vi "10 - colour keying.vi"() -> ()   [LabVIEW 2015]
uses:
  Libraries/LibSDL2 Wrapper/Controls/Init Flags.ctl
  Libraries/LibSDL2 Wrapper/Controls/NULL.ctl
  Libraries/LibSDL2 Wrapper/Controls/Rectangle.ctl
  Libraries/LibSDL2 Wrapper/Controls/RGB.ctl
  Libraries/LibSDL2 Wrapper/LibSDL2.lvlib
  Libraries/LibSDL2_Image Wrapper/LibSDL2_Image.lvlib
  Libraries/SDL2 Utility/SDL2 Utility.lvlib
panel:
  out "Error":string
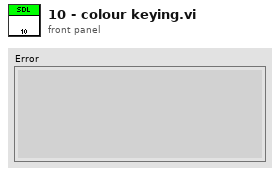
[diagram p1: front panel]
types:
  T1 = typedef "LibSDL2.lvlib/RGB.ctl" = cluster{"R":u8, "G":u8, "B":u8}
  T2 = typedef "LibSDL2.lvlib/Rectangle.ctl" = cluster{"x":i32, "y":i32, "Width":i32, "Height":i32}
  T3 = typedef "LibSDL2.lvlib/NULL.ctl" = enum32{"NULL"}
  T4 = typedef "LibSDL2.lvlib/Init Flags.ctl" = u32
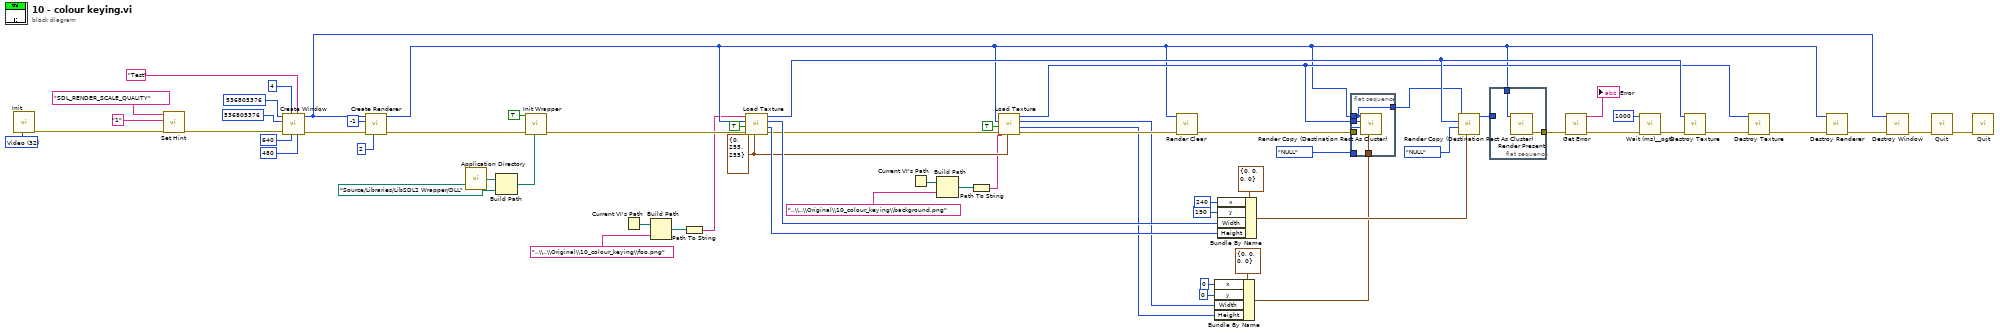
[diagram p0: block diagram]
diagram:
  w18 = T1 {"R"=0, "G"=255, "B"=255} ("RGB")
  w64 = T4 32 items=["Timer"=1, "Audio"=16, "Video"=32, "Joystick"=512, "Haptic"=4096, "Game Controller"=8192, "Events"=16384, "No Parachute"=1048576, "Everything"=17244689] ("Init Flags")
  n1 = call "Init.vi"("Flags"=w64) -> ("error out"=w52:errorcluster)  [unwired: 9 in, 1 out]
  n2 = call "Set Hint.vi"("error in"=w52, "Value"="1", "Name"="SDL_RENDER_SCALE_QUALITY") -> ("error out"=w51:errorcluster)  [unwired: 7 in, 1 out]
  n3 = call "Create Window.vi"("Height"=480, "Title"="Test", "Width"=640, "Flags"=u32 4, "error in"=w51, "Position y"=u32 536805376 ("Flags"), "Position x"=u32 536805376 ("Flags")) -> ("error out"=w48:errorcluster, "Window Pointer"=w39:u32)  [unwired: 3 in]
  n4 = call "Create Renderer.vi"("Flags"=u32 2, "error in"=w48, "Index"=-1, "Window Pointer"=w39) -> ("error out"=w16:errorcluster, "Renderer Pointer"=w14:u32)  [unwired: 6 in]
  n5 = call <vilib>:"Application Directory.vi"() -> ("Application Directory"=w11:path)
  n6 = Build Path(base path=w11, name or relative path=path "Source/Libraries/LibSDL2 Wrapper/DLL" ("DLL Directory")) -> (appended path=w9:path)
  n7 = call "Init Wrapper.vi"("DLL Directory"=w9, "error in"=w16, "PNG (F)"=TRUE ("PNG")) -> ("error out"=w17:errorcluster)  [unwired: 7 in, 1 out]
  n8 = Current VI's Path() -> (path=w8:path)
  n9 = Build Path(base path=w8, name or relative path="..\\..\\Original\\10_colour_keying\\foo.png" ("File")) -> (appended path=w7:path)
  n10 = Path To String(path=w7) -> (string=w5:string)
  n11 = call "Load Texture.vi"("RGB"=w18, "error in"=w17, "Apply Colour Key (F)"=TRUE, "Renderer Pointer"=w14, "File"=w5) -> ("error out"=w31:errorcluster, "Height"=w33:i32, "Width"=w34:i32, "Optimised Texture Pointer"=w24:u32)  [unwired: 3 in]
  n12 = Current VI's Path() -> (path=w2:path)
  n13 = Build Path(base path=w2, name or relative path="..\\..\\Original\\10_colour_keying\\background.png" ("File")) -> (appended path=w3:path)
  n14 = Path To String(path=w3) -> (string=w1:string)
  n15 = call "Load Texture.vi"("RGB"=w18, "error in"=w31, "Apply Colour Key (F)"=TRUE, "Renderer Pointer"=w14, "File"=w1) -> ("error out"=w30:errorcluster, "Height"=w19:i32, "Width"=w20:i32, "Optimised Texture Pointer"=w22:u32)  [unwired: 3 in]
  n16 = call "Render Clear.vi"("error in"=w30, "Renderer Pointer"=w14) -> ("error out"=w15:errorcluster)  [unwired: 8 in, 1 out]
  n17 = Bundle By Name(cluster=T2 {"x"=0, "y"=0, "Width"=0, "Height"=0} ("Destination Rectangle"), "x"=0, "y"=0, "Width"=w20, "Height"=w19) -> (w25:T2)
  n18 = Bundle By Name(cluster=T2 {"x"=0, "y"=0, "Width"=0, "Height"=0} ("Destination Rectangle"), "x"=240, "y"=190, "Width"=w34, "Height"=w33) -> (w37:T2)
  n19 = flat-sequence {
    tunnel: NULL."NULL" ("Null") -> [w68]
    tunnel: w25 -> [w67]
    tunnel: w14 -> [w65]
    tunnel: w22 -> [w66]
    tunnel: w15 -> [_]
    tunnel: [w65] -> w13
    frame #0 {
      n20 = call "Render Copy (Destination Rect As Cluster).vi"("Destination Rectangle"=w67, "Source Rectangle Pointer"=w68, "Texture Pointer"=w66, "Renderer Pointer"=w65) -> ()  [unwired: 7 in, 1 out]
    }
  }
  n21 = call "Render Copy (Destination Rect As Cluster).vi"("Destination Rectangle"=w37, "Source Rectangle Pointer"=NULL."NULL" ("Null"), "Texture Pointer"=w24, "Renderer Pointer"=w13) -> ("Return"=w12:i32)  [unwired: 7 in]
  n22 = flat-sequence {
    tunnel: [w70] -> w43
    tunnel: w14 -> [w69]
    tunnel: w12 -> [_]
    frame #0 {
      n23 = call "Render Present.vi"("Renderer Pointer"=w69) -> ("error out"=w70:errorcluster)  [unwired: 10 in]
    }
  }
  n24 = call "Get Error.vi"("error in"=w43) -> ("error out"=w42:errorcluster, "Error"=→"Error":string)  [unwired: 9 in]
  n25 = call <userlib>:"Wait (ms)__ogtk.vi"("error in (no error)"=w42, "milliseconds to wait"=u32 1000) -> ("error out"=w45:errorcluster)  [unwired: 8 in, 1 out]
  n26 = call "Destroy Texture.vi"("error in"=w45, "Texture Pointer"=w24) -> ("error out"=w23:errorcluster)  [unwired: 9 in]
  n27 = call "Destroy Texture.vi"("error in"=w23, "Texture Pointer"=w22) -> ("error out"=w21:errorcluster)  [unwired: 9 in]
  n28 = call "Destroy Renderer.vi"("error in"=w21, "Renderer Pointer"=w14) -> ("error out"=w44:errorcluster)  [unwired: 9 in]
  n29 = call "Destroy Window.vi"("error in"=w44, "Window Pointer"=w39) -> ("error out"=w55:errorcluster)  [unwired: 9 in]
  n30 = call "Quit.vi"("error in"=w55) -> ("error out"=w54:errorcluster)  [unwired: 10 in]
  n31 = call "Quit.vi"("error in"=w54) -> ()  [unwired: 10 in, 1 out]
